vi "image to array develop.vi"() -> ()   [LabVIEW 2023]
panel:
  out "String":string
  out "Array":u8[][](array[numeric])
  out "Image":T1(plugin-control)
  out "Image Name":string="image"
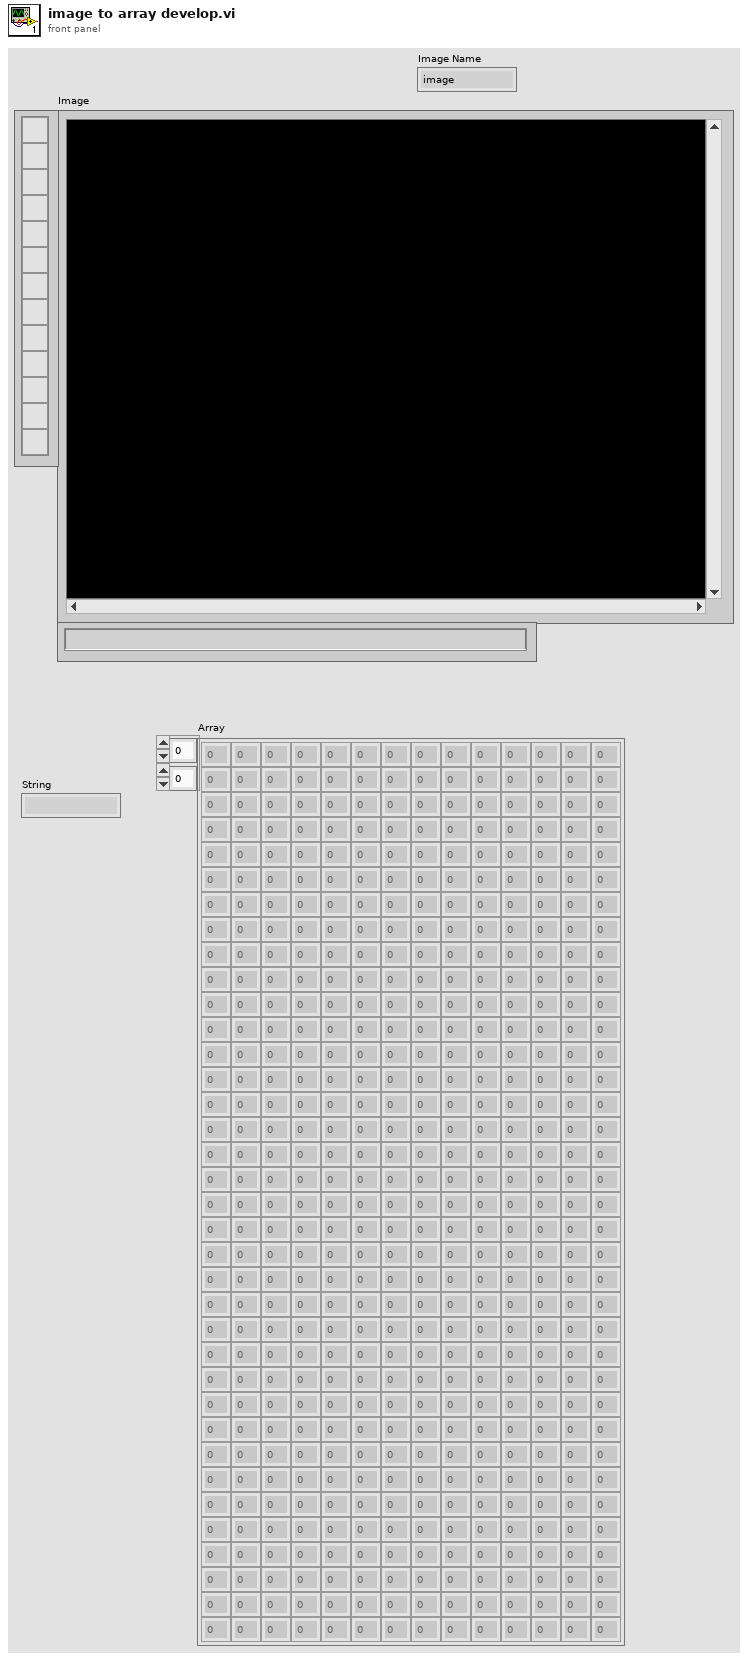
[diagram p1: front panel]
types:
  T1 = typedef "IMAQ Image.ctl" = refnum<image>
  T2 = typedef "Image Type" = u32
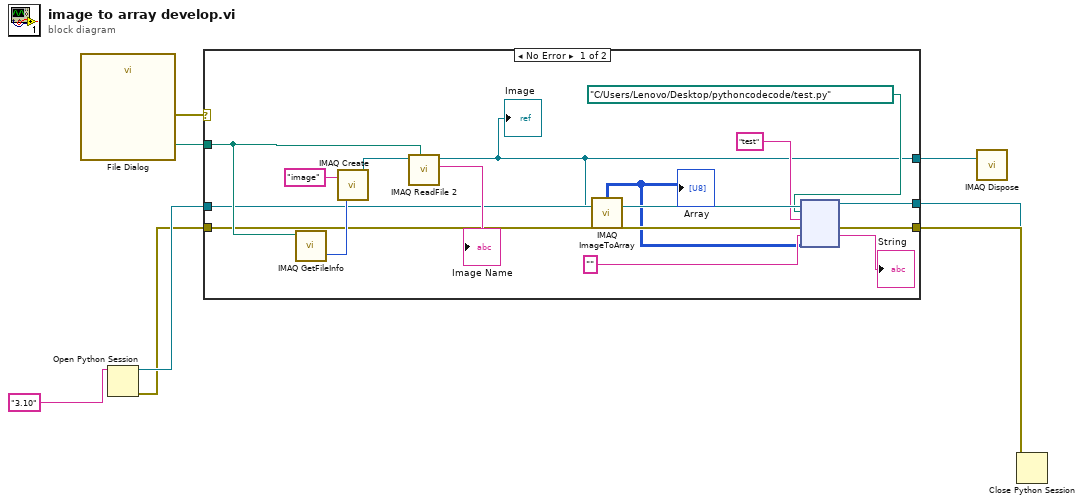
[diagram p0: block diagram]
diagram:
  n1 = call "File Dialog"() -> ("selected path"=w8:path, "error out"=w7:errorcluster)  [unwired: 12 in, 2 out]
  n2 = Open Python Session(python version="3.10") -> (session out=w5:refnum<k35>, error out=w4:errorcluster)  [unwired: 2 in]
  n3 = case shown="No Error" w7 {
    tunnel: w8 -> [w21 _]
    tunnel: w5 -> [w18 _]
    tunnel: w4 -> [w17 _]
    tunnel: [w16 _] -> w3
    tunnel: [w15 _] -> w2
    tunnel: [w9 _] -> w1
    frame No Error {
      n4 = call "IMAQ GetFileInfo"("File Path"=w21) -> ("Image Type"=w20:T2)  [unwired: 4 in, 6 out]
      n5 = call "IMAQ Create"("Image Name"="image", "Image Type"=w20) -> ("New Image"=w22:T1)  [unwired: 3 in, 1 out]
      n6 = call "IMAQ ReadFile 2"("File Path"=w21, "Image"=w22) -> ("File Type out"=→"Image Name":string, "Image Out"=w9:T1)  [unwired: 5 in, 3 out]
      "Image" <- w9
      n7 = call "IMAQ ImageToArray"("Image"=w9) -> ("Image Pixels (U8)"=w13:u8[][])  [unwired: 3 in, 4 out]
      "Array" <- w13
      n8 = node(w18, path "C:/Users/Lenovo/Desktop/pythoncodecode/test.py" ("Path"), "test", w17, "", w13) -> (w15:refnum<k35>, w16:errorcluster, →"String":string)  [unwired: 1 in, 2 out]
    }
    frame Error {
    }
  }
  n9 = call "IMAQ Dispose"("Image"=w1) -> ()  [unwired: 5 in, 1 out]
  n10 = Close Python Session(session in=w2, error in=w3) -> ()  [unwired: 1 out]
